vi "NF90 run.vi"(8 "Error In":errorcluster, 11 "port number in":refnum<visa-resource-name>) -> (0 "Error Out":errorcluster, 1 "killed":bool, 3 "port number out":refnum<visa-resource-name>)   [LabVIEW 2019]
uses:
  NF90 commands.ctl
  Kill.ctl
panel:
  in  "quit":bool
  in  "Stop":bool
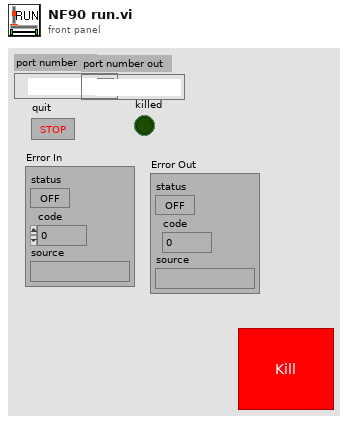
[diagram p1: front panel]
types:
  T1 = typedef "NF90 commands.ctl" = enum16{"Index", "Speed", "Acceleration", "Backlash", "Quit", "Run", "Null indexes", "Verify status", "Clear program", "Computer Control", "Go", "Put Controller on Hold", "Position"}
  T2 = typedef "Kill.ctl" = enum16{"Kill", "Decelerate"}
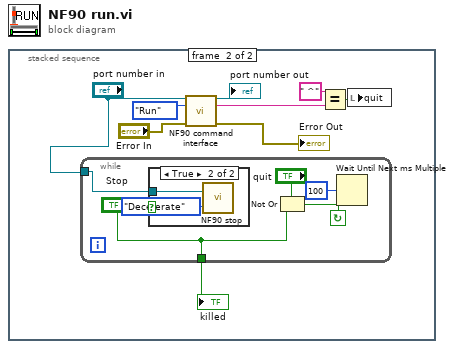
[diagram p0: block diagram]
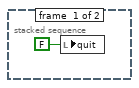
[diagram p2: hidden frame]
diagram:
  n1 = stacked-sequence {
    frame #0 {
      n2 = local write "quit"(FALSE ("quit")) -> ()
    }
    frame #1 {
      n3 = while {
        tunnel: ["Stop"] -> w5
        tunnel: "port number in" -> [w15]
        stop <- w14 continue-if-true
        n4 = case shown="True" "Stop" {
          tunnel: w15 -> [_ w17]
          frame False {
          }
          frame True {
            n5 = call "NF90 stop.vi"("Stop"=Kill."Decelerate", "port number"=w17) -> ()  [unwired: 2 in]
          }
        }
        n6 = Not Or(1:"Stop", 2:"quit") -> (0:w14:bool)
        n7 = Wait Until Next ms Multiple(millisecond multiple=u32 100) -> ()  [unwired: 1 out]
      }
      "killed" <- w5
      n8 = call "NF90 command interface.vi"("port number in"="port number in", "commands"=NF90_commands."Run", "Error In"="Error In") -> ("port number out"=→"port number out":refnum<visa-resource-name>, "Response"=w8:string, "Error Out"=→"Error Out":errorcluster)  [unwired: 8 in, 2 out]
      n9 = Equal?(x=w8, y=" ^") -> (x = y?=w2:bool)
      n10 = local write "quit"(w2) -> ()
    }
  }
